vi "test-Encrypt (FFT - mismatch Multiplier).vi"(8 "error in (no error)":errorcluster, 11 "TestCase in":refnum<class "Test Argument Encryption.lvclass">) -> (0 "error out":errorcluster, 3 "TestCase out":refnum<class "Test Argument Encryption.lvclass">)   [LabVIEW 2019, in "Test Argument Encryption.lvclass"]
uses:
  Test Argument Encryption.lvclass
  C:/Program Files/National Instruments/LabVIEW 2024/vi.lib/Astemes/LUnit/Test Case.lvclass
  Encryption/FFT/FFT.lvclass
  C:/Development/Open Source/tsc-event-logger/Encryption/Encryption.lvclass
  <vilib>/Astemes/LUnit/Test Case.lvclass/Test Case.ctl
  87440836-0619-4db8-af71-0960f7dd8b4a.vi
  <vilib>/Astemes/LUnit/Core/LUnit Test Case/Private/Append Pass Result.vi
  <vilib>/Astemes/LUnit/Core/LUnit Test Case/Private/Append Fail Result.vi
  87440836-0619-4db8-af71-0960f7dd8b4a.vi/9c5d11cd-9439-4240-a1ee-d9baace9c924.vi
  <vilib>/Astemes/LUnit/Core/LUnit Test Case/Private/Run In UI.vi
  <vilib>/Utility/error.llb/Clear Errors.vi
  Encryption/Encryption.lvclass
  Layouts/Layout.lvclass
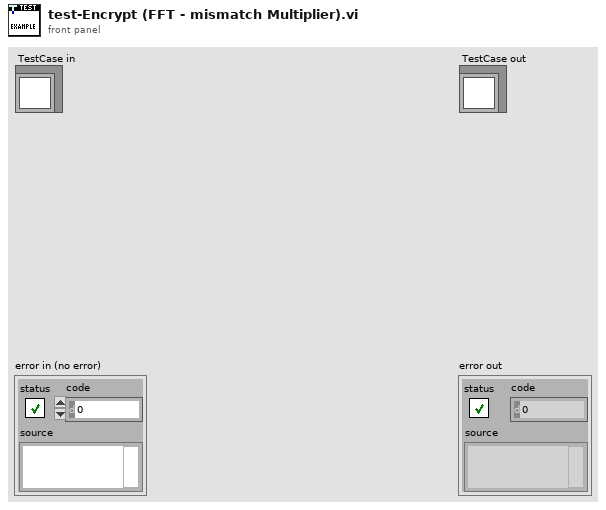
[diagram p1: front panel]
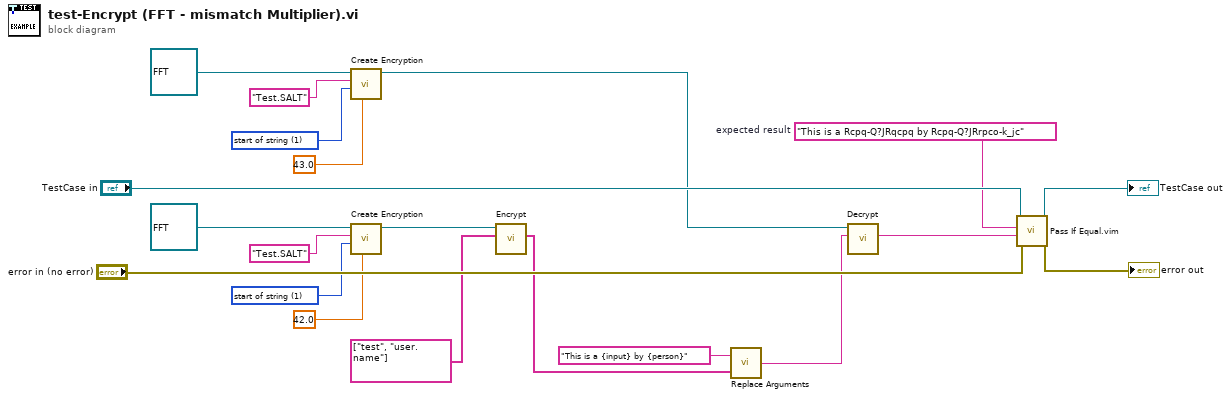
[diagram p0: block diagram]
diagram:
  w4 = u16 1 items=["both", "start of string", "end of string"] ("SALT location (start of string)")
  w13 = u16 1 items=["both", "start of string", "end of string"] ("SALT location (start of string)")
  w16 = "This is a Rcpq-Q?JRqcpq by Rcpq-Q?JRrpco-k_jc"  # expected result
  n1 = call "Create Encryption.vi"("Multiplier"=43.0, "SALT location (start of string)"=w4, "SALT"="Test.SALT", "Encryption Method"=refnum<class "FFT.lvclass"> refnum ("TSC Event Logger.lvlib:FFT.lvclass")) -> ("Encryption output"=w1:refnum<class "FFT.lvclass">)  [unwired: 6 in, 1 out]
  n2 = call "Create Encryption.vi"("Multiplier"=42.0, "SALT location (start of string)"=w13, "SALT"="Test.SALT", "Encryption Method"=refnum<class "FFT.lvclass"> refnum ("TSC Event Logger.lvlib:FFT.lvclass")) -> ("Encryption output"=w11:refnum<class "FFT.lvclass">)  [unwired: 6 in, 1 out]
  n3 = call-dynamic "Encrypt.vi"("Arguments"=string[] ["test", "user.name"], "FFT in"=w11) -> ("Encrypted Arguments"=w8:string[])  [unwired: 7 in, 2 out]
  n4 = call "Replace Arguments.vi"("Arguments"=w8, "Message"="This is a {input} by {person}") -> ("Output Message"=w7:string)
  n5 = call-dynamic "Decrypt.vi"("Message"=w7, "FFT in"=w1) -> ("Decrypted Message"=w6:string)  [unwired: 7 in, 2 out]
  n6 = call "Pass If Equal.vim"("error in (no error)"="error in (no error)", "Actual"=w6, "Expected"=w16, "LUnit Test Case In"="TestCase in") -> ("error out"=→"error out":errorcluster, "LUnit Test Case Out"=→"TestCase out":refnum<class "Test Argument Encryption.lvclass">)  [unwired: 6 in]
